vi "Get as Waveform.vi"(8 "error in (no error)":errorcluster, 10 "Name Array":string[](array[string]), 11 "JSON Value In":refnum<class "JSON Value.lvclass">) -> (0 "error out":errorcluster, 2 "Waveform":waveform(dbl), 3 "JSON Value Out":refnum<class "JSON Value.lvclass">)   [LabVIEW 2011, in "JSON Object.lvclass"]
doc: "Gets a JSON object from a JSON collection by it's path (an array of strings).\n\nCopyright 2012 James David Powell, Shaun Rumbell and Ton Plomp\nMore information on http://lavag.org/topic/16217-cr-json-labview"
uses:
  JSON Object/JSON Object.lvclass
  JSON Value.lvclass
  JSON Scalar/Get as Timestamp.vi
  JSON Scalar/Get as DBL.vi
  JSON Array/Get Array.vi
  Get Polymorphic/JSON GetSet.lvlib
  JSON Scalar/JSON Scalar.lvclass
  JSON Array/JSON Array.lvclass
  Get sub-Item by names.vi
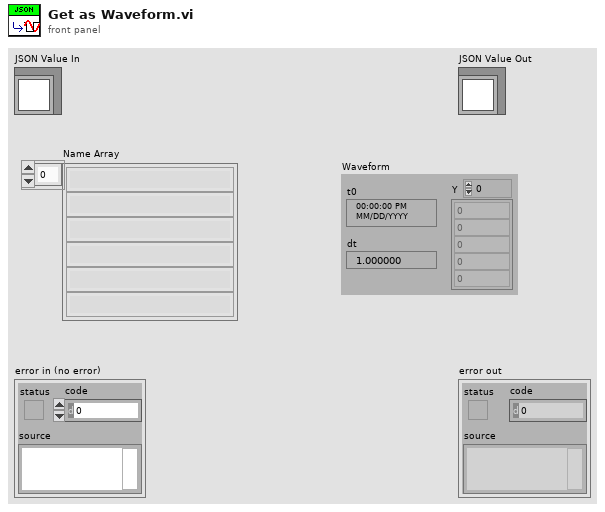
[diagram p1: front panel]
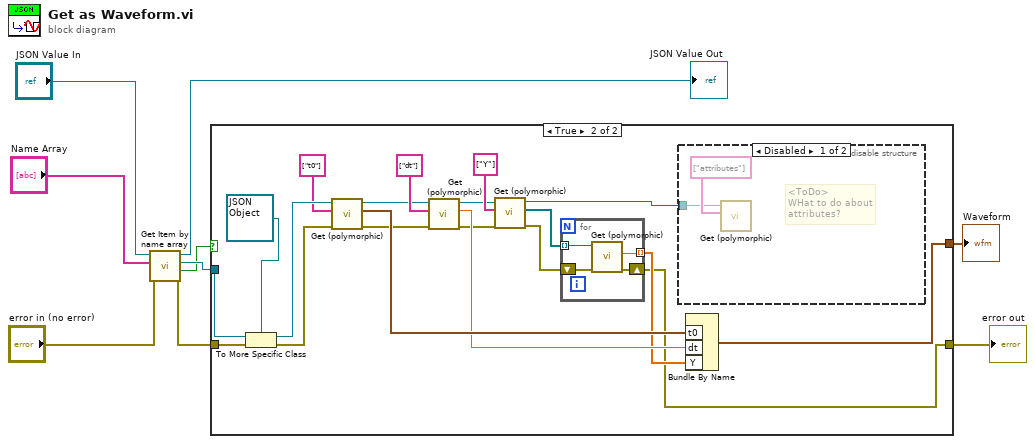
[diagram p0: block diagram]
diagram:
  n1 = call "Get Item by name array.vi"("error in (no error)"="error in (no error)", "Name Array"="Name Array", "JSON Value In"="JSON Value In") -> ("error out"=w3:errorcluster, "found"=w4:bool, "Value"=w5:refnum<class "JSON Value.lvclass">, "JSON Value Out"=→"JSON Value Out":refnum<class "JSON Value.lvclass">)  [unwired: 5 in]
  n2 = case shown="True" w4 {
    tunnel: w5 -> [_ w30]
    tunnel: w3 -> [w10 w29]
    tunnel: [w10 w11] -> w2
    tunnel: [_ w16] -> w1
    frame False {
    }
    frame True {
      n3 = To More Specific Class(target class=refnum<class "JSON Object.lvclass"> refnum ("JSON Object.lvclass"), reference=w30, error in=w29) -> (specific class reference=w27:refnum<class "JSON Object.lvclass">, error out=w15:errorcluster)
      n4 = call-poly "Get (polymorphic).vi"("error in (no error)"=w15, "Name Array"=string[] ["t0"], "JSON Value in"=w27) -> ("error out"=w14:errorcluster, "Time Stamp"=w25:timestamp, "JSON Value out"=w23:refnum<class "JSON Object.lvclass">)  [unwired: 6 in]
      n5 = call-poly "Get (polymorphic).vi"("error in (no error)"=w14, "Name Array"=string[] ["dt"], "JSON Value in"=w23) -> ("error out"=w13:errorcluster, "Number"=w22:dbl, "JSON Value out"=w20:refnum<class "JSON Object.lvclass">)  [unwired: 6 in]
      n6 = call-poly "Get (polymorphic).vi"("error in (no error)"=w13, "Name Array"=string[] ["Y"], "JSON Array in"=w20) -> ("error out"=w12:errorcluster, "Array"=w19:refnum<class "JSON Value.lvclass">[], "JSON Array out"=w17:refnum<class "JSON Object.lvclass">)  [unwired: 6 in]
      n7 = for {
        tunnel: w19 -> [w36] mode=indexing
        tunnel: [w35] -> w18 mode=indexing
        shift-right: [w33] -> w11
        shift-left: w12 -> [w34]
        n8 = call-poly "Get (polymorphic).vi"("error in (no error)"=w34, "JSON Value in"=w36) -> ("error out"=w33:errorcluster, "Number"=w35:dbl)  [unwired: 7 in, 1 out]
      }
      n9 = disable-structure shown="Disabled" {
        disable-tunnel: w17 -> [w31 _]
        frame Disabled {
          # "<ToDo>\nWHat to do about\nattributes?"
          n10 = call-poly "Get (polymorphic).vi"("Name Array"=string[] ["attributes"], "JSON Value In"=w31) -> ()  [unwired: 6 in, 4 out]
        }
        frame Enabled {
        }
      }
      n11 = Bundle By Name("t0"=w25, "dt"=w22, "Y"=w18) -> (w16:waveform(dbl))  [unwired: 1 in]
    }
  }
  "error out" <- w2
  "Waveform" <- w1
